vi "Parse (Orientation Update Matrix).vi"(7 "Message In":string) -> (6 "Orientation Update Matrix":sgl[][](array[numeric]), 15 "Timer":u32)   [LabVIEW 2012, in "MicroStrain 3DM-GXx.lvlib"]
doc: "Parse the data from the 0xC6 message into the Orientation Update Matrix. This is a 9 component coordinate transformation matrix which describes the change in orientation of the device during the period of the most recent calculation cycle."
uses:
  <instrlib>/MicroStrain 3DM-GXx/MicroStrain 3DM-GXx.lvlib
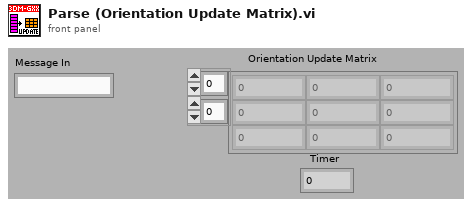
[diagram p1: front panel]
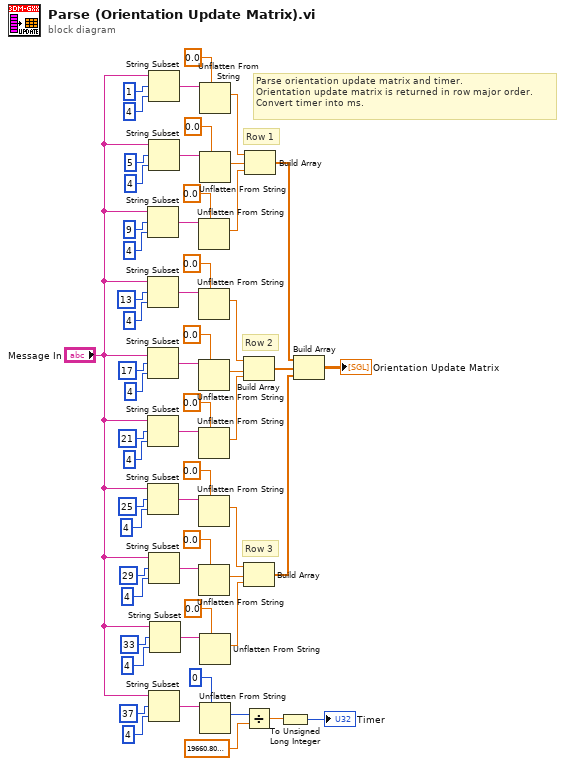
[diagram p0: block diagram]
diagram:
  # "Parse orientation update matrix and timer.\nOrientation update matrix is returned in row major order.\nConvert timer into ms."
  # "Row 3"
  # "Row 2"
  # "Row 1"
  n1 = String Subset(string="Message In", offset (0)=9, length (rest)=4 ("length (rest)")) -> (substring=w48:string)
  n2 = String Subset(string="Message In", offset (0)=13, length (rest)=4 ("length (rest)")) -> (substring=w45:string)
  n3 = String Subset(string="Message In", offset (0)=17, length (rest)=4 ("length (rest)")) -> (substring=w40:string)
  n4 = String Subset(string="Message In", offset (0)=21, length (rest)=4 ("length (rest)")) -> (substring=w37:string)
  n5 = String Subset(string="Message In", offset (0)=25, length (rest)=4 ("length (rest)")) -> (substring=w32:string)
  n6 = String Subset(string="Message In", offset (0)=1, length (rest)=4 ("length (rest)")) -> (substring=w56:string)
  n7 = String Subset(string="Message In", offset (0)=5, length (rest)=4 ("length (rest)")) -> (substring=w53:string)
  n8 = String Subset(string="Message In", offset (0)=29, length (rest)=4 ("length (rest)")) -> (substring=w23:string)
  n9 = String Subset(string="Message In", offset (0)=37, length (rest)=4 ("length (rest)")) -> (substring=w15:string)
  n10 = String Subset(string="Message In", offset (0)=33, length (rest)=4 ("length (rest)")) -> (substring=w18:string)
  n11 = Unflatten From String(type=sgl 0.0, binary string=w48) -> (value=w28:sgl)  [unwired: 3 in, 2 out]
  n12 = Unflatten From String(type=sgl 0.0, binary string=w45) -> (value=w26:sgl)  [unwired: 3 in, 2 out]
  n13 = Unflatten From String(type=sgl 0.0, binary string=w40) -> (value=w27:sgl)  [unwired: 3 in, 2 out]
  n14 = Unflatten From String(type=sgl 0.0, binary string=w37) -> (value=w25:sgl)  [unwired: 3 in, 2 out]
  n15 = Unflatten From String(type=sgl 0.0, binary string=w32) -> (value=w11:sgl)  [unwired: 3 in, 2 out]
  n16 = Unflatten From String(type=sgl 0.0, binary string=w23) -> (value=w12:sgl)  [unwired: 3 in, 2 out]
  n17 = Unflatten From String(type=sgl 0.0, binary string=w56) -> (value=w29:sgl)  [unwired: 3 in, 2 out]
  n18 = Unflatten From String(type=sgl 0.0, binary string=w53) -> (value=w30:sgl)  [unwired: 3 in, 2 out]
  n19 = Unflatten From String(type=sgl 0.0, binary string=w18) -> (value=w10:sgl)  [unwired: 3 in, 2 out]
  n20 = Unflatten From String(type=u32 0, binary string=w15) -> (value=w6:u32)  [unwired: 3 in, 2 out]
  n21 = Build Array(w26, w27, w25) -> (w4:sgl[])
  n22 = Build Array(w11, w12, w10) -> (w2:sgl[])
  n23 = Divide(x=w6, y=sgl 19660.8) -> (x/y=w5:sgl)
  n24 = Build Array(w29, w30, w28) -> (w3:sgl[])
  n25 = To Unsigned Long Integer(number=w5) -> (unsigned 32bit integer=→"Timer":u32)
  n26 = Build Array(w3, w4, w2) -> (→"Orientation Update Matrix":sgl[][])
